vi "Set User.vi"(8 "error in (no error)":errorcluster, 10 "User":refnum<class "User.lvclass">, 11 "Processing in":refnum<class "Processing.lvclass">) -> (0 "error out":errorcluster, 3 "Processing out":refnum<class "Processing.lvclass">)   [LabVIEW 2020, in "HTTP Server.lvlib" / "Processing.lvclass"]
uses:
  Processing.lvclass
  Security/Security.lvclass
  Values/Values.lvclass
  User/User.lvclass
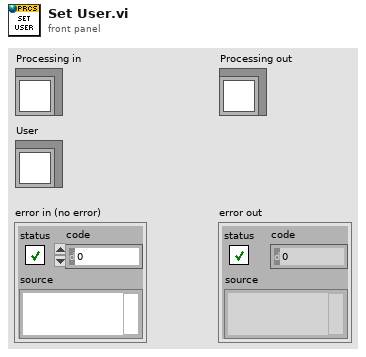
[diagram p1: front panel]
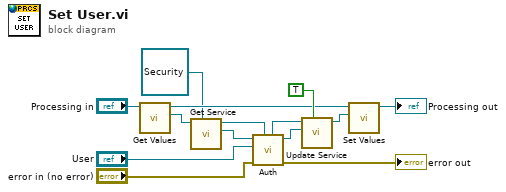
[diagram p0: block diagram]
diagram:
  n1 = call "Get Values.vi"("Processing in"="Processing in") -> ("Values"=w3:refnum<class "Values.lvclass">, "Processing out"=w12:refnum<class "Processing.lvclass">)  [unwired: 9 in]
  n2 = call "Get Service.vi"("Service Type"=refnum<class "Security.lvclass"> refnum ("Security in"), "Values in"=w3) -> ("Service"=w1:refnum<class "Security.lvclass">, "Values out"=w4:refnum<class "Values.lvclass">)  [unwired: 7 in, 1 out]
  n3 = call "Auth.vi"("Values In"=w4, "error in (no error)"="error in (no error)", "User (None)"="User", "Security in"=w1) -> ("error out"=→"error out":errorcluster, "Security out"=w14:refnum<class "Security.lvclass">, "Values"=w10:refnum<class "Values.lvclass">)  [unwired: 5 in]
  n4 = call "Update Service.vi"("Overwrite? (F)"=TRUE, "Service"=w14, "Values in"=w10) -> ("Values out"=w11:refnum<class "Values.lvclass">)  [unwired: 7 in, 1 out]
  n5 = call "Set Values.vi"("Values"=w11, "Processing in"=w12) -> ("Processing out"=→"Processing out":refnum<class "Processing.lvclass">)  [unwired: 9 in]
